vi "Serial Print Target IP.vi"(7 "WiFi Mode":T1(ring)=enum."WIFI_AP", 8 "Error In":errorcluster) -> (0 "Error Out":errorcluster)   [LabVIEW 2014, in "ESP8266 WiFi Wrapper.lvlib"]
uses:
  <vilib>/Aledyne-TSXperts/Arduino Compatible Compiler for LabVIEW/addons/ESP8266 WiFi Wrapper/ESP8266 WiFi Wrapper.lvlib
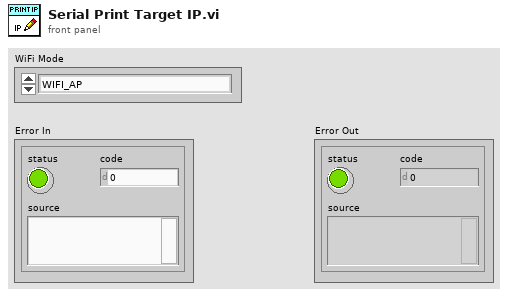
[diagram p1: front panel]
types:
  T1 = enum16{"WIFI_OFF", "WIFI_STA", "WIFI_AP", "WIFI_AP_STA"}
  T2 = enum8{"WIFI_OFF", "WIFI_STA", "WIFI_AP", "WIFI_AP_STA"}
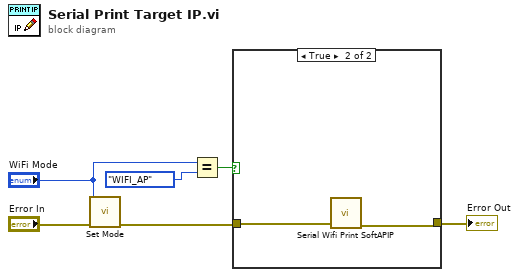
[diagram p0: block diagram]
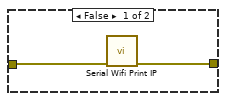
[diagram p2: hidden frame]
diagram:
  n1 = call <vilib>:"Set Mode.vi"("Error In"="Error In", "WiFi Server Mode"="WiFi Mode") -> ("Error Out"=w6:errorcluster)  [unwired: 9 in]
  n2 = Equal?(x="WiFi Mode", y=T2."WIFI_AP" ("Enum")) -> (x = y?=w1:bool)
  n3 = case shown="True" w1 {
    tunnel: w6 -> [w8 w10]
    tunnel: [w7 w9] -> w4
    frame False {
      n4 = call <vilib>:"Serial Wifi Print IP.vi"("Error In"=w8) -> ("Error Out"=w7:errorcluster)  [unwired: 10 in]
    }
    frame True {
      n5 = call <vilib>:"Serial Wifi Print SoftAPIP.vi"("Error In"=w10) -> ("Error Out"=w9:errorcluster)  [unwired: 10 in]
    }
  }
  "Error Out" <- w4
